vi "Keithley 6514 Coulombs Config.vi"(0 "Resource In":refnum<visa-resource-name>, 1 "Check For SCPI Errors? (T)":bool=TRUE, 5 "NPLC value (1.00)":sgl=1.0 min=0.01 max=10 step=0.01 format="%.2f", 7 "range (autorange:0)":u16(ring) items=["autorange", "set min range", "set max range", "set range value"], 9 "range value (amps) (2.1e-6)":sgl=2.101e-06 min=0 max=2.1e-05 step=1.1e-08 format="%^.2e", 11 "error in (no error)":T1, 12 "AutoRange Limit (HIGH:T)":bool=TRUE, 13 "AutoDischarge Level (2e-6)":sgl=2e-06 min=-2.1e-05 max=2.1e-05 step=1e-12 format="%^.6e", 14 "AutoDischarge State (OFF:F)":bool) -> (4 "Resource Out (dupl)":refnum<visa-resource-name>, 15 "error out":T1)   [LabVIEW 2009, in "Keithley 6514 LV 2009.lvlib"]
doc: "This VI is used to configure the settings for charge measurements. The instrument can be in any mode when this VI is run. The settings will go into effect and the instrument will go into the charge mode.\n\nNPLC Value:\n0.01 to 10\n\nRange:\n0 = Autorange\n1 = set minimum range\n2 = set maximum range\n3 = set range by value\n\nrange value:\n0 to 21e-6\n\nAutorange Limit:\nTRUE = HIGH\nFALSE = LOW\n\nAutoDischarge Level:\n-21e-6 to 21e6\n\nAutoDischarge State:\nTRUE=ON\nFALSE = OFF"
uses:
  Keithley 6514 LV 2009.lvlib
panel:
  # "HIGH\nLOW"
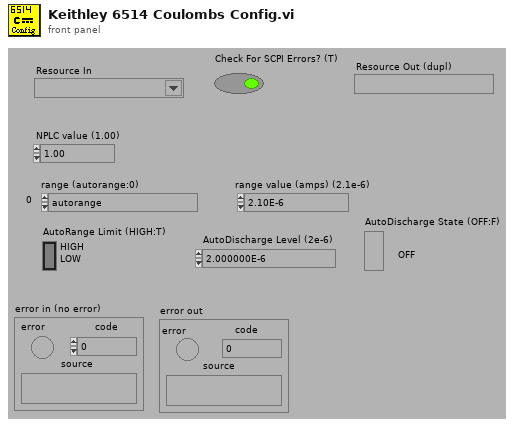
[diagram p1: front panel]
types:
  T1 = cluster{"error":bool, "code":i32, "source":string}
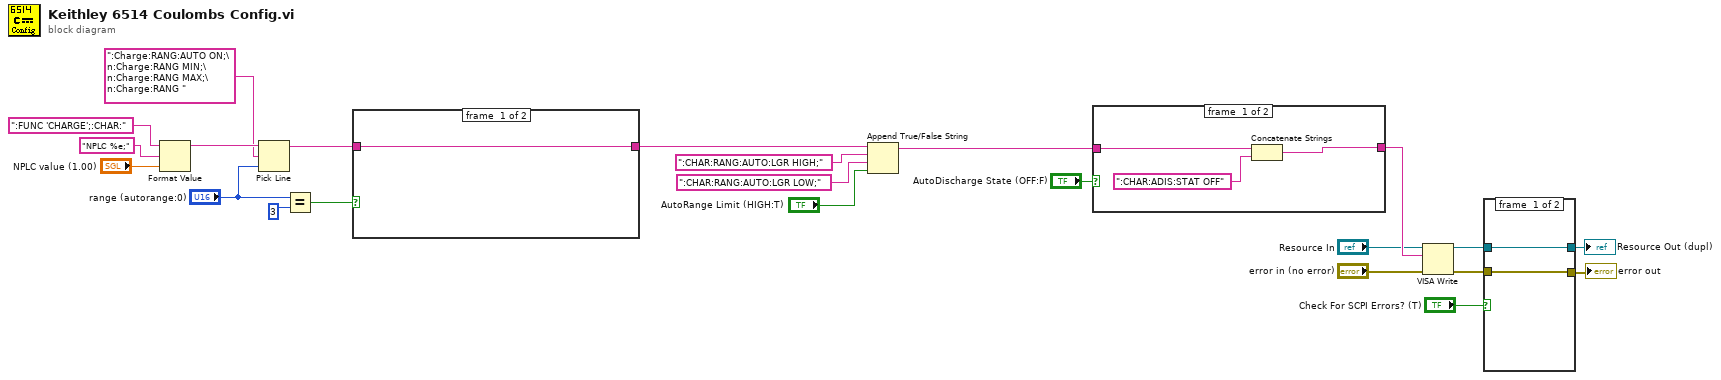
[diagram p0: block diagram]
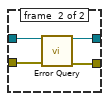
[diagram p2: hidden frame]
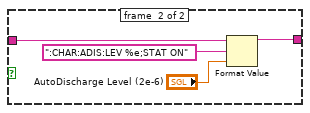
[diagram p3: hidden frame]
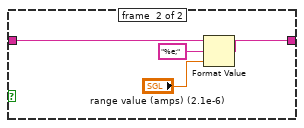
[diagram p4: hidden frame]
diagram:
  n1 = Format Value(string ("")=":FUNC 'CHARGE';:CHAR:", format string="NPLC %e;", value (0)="NPLC value (1.00)") -> (output string=w13:string)
  n2 = Pick Line(string ("")=w13, multi-line string=":Charge:RANG:AUTO ON;\n:Charge:RANG MIN;\n:Charge:RANG MAX;\n:Charge:RANG ", line index="range (autorange:0)") -> (output string=w11:string)
  n3 = Equal?(x="range (autorange:0)", y=u16 3) -> (x = y?=w23:bool)
  n4 = case shown="False" w23 {
    tunnel: w11 -> [w24 w27]
    tunnel: [w24 w25] -> w10
    frame #0 {
    }
    frame #1 {
      n5 = Format Value(string ("")=w27, format string="%e;", value (0)="range value (amps) (2.1e-6)") -> (output string=w25:string)
    }
  }
  n6 = Append True/False String(1:"AutoRange Limit (HIGH:T)", 2:":CHAR:RANG:AUTO:LGR LOW;", 3:":CHAR:RANG:AUTO:LGR HIGH;", 4:w10) -> (0:w9:string)
  n7 = case shown="True" "AutoDischarge State (OFF:F)" {
    tunnel: [w30 w35] -> w8
    tunnel: w9 -> [w29 w32]
    frame #0 {
      n8 = Concatenate Strings(w29, ":CHAR:ADIS:STAT OFF") -> (w30:string)
    }
    frame #1 {
      n9 = Format Value(string ("")=w32, format string=":CHAR:ADIS:LEV %e;STAT ON", value (0)="AutoDischarge Level (2e-6)") -> (output string=w35:string)
    }
  }
  n10 = VISA Write(VISA resource name="Resource In", write buffer=w8, error in (no error)="error in (no error)") -> (VISA resource name out=w4:refnum<visa-resource-name>, error out=w3:errorcluster)  [unwired: 1 out]
  n11 = case shown="False" "Check For SCPI Errors? (T)" {
    tunnel: w4 -> [w37 w41]
    tunnel: w3 -> [w36 w40]
    tunnel: [w37 w39] -> w2
    tunnel: [w36 w38] -> w1
    frame #0 {
    }
    frame #1 {
      n12 = call "Error Query.vi"("VISA Resource In"=w41, "error in (no error)"=w40) -> ("VISA Resource Out (dupl)"=w39:refnum<visa-resource-name>, "error out"=w38:errorcluster)  [unwired: 10 in, 2 out]
    }
  }
  "error out" <- w1
  "Resource Out (dupl)" <- w2
